vi "Date.vi"(11 "Output All":string) -> (3 "Date":string)   [LabVIEW 2015]
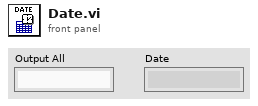
[diagram p1: front panel]
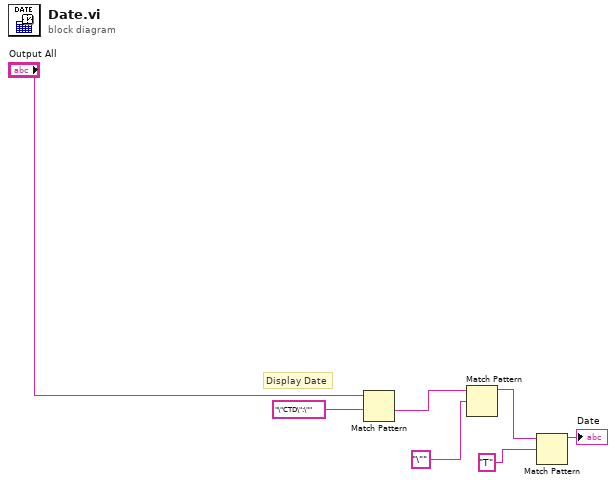
[diagram p0: block diagram]
diagram:
  # "Display Date"
  n1 = Match Pattern(string="Output All", regular expression="\"CTD\":\"") -> (after substring=w1:string)  [unwired: 1 in, 3 out]
  n2 = Match Pattern(string=w1, regular expression="\"") -> (before substring=w4:string)  [unwired: 1 in, 3 out]
  n3 = Match Pattern(string=w4, regular expression="T") -> (before substring=→"Date":string)  [unwired: 1 in, 3 out]
